vi "Obtain Request Events.vi"(8 "error in":errorcluster, 10 "Create New? (F)":bool) -> (0 "error out":errorcluster, 2 "EL72xx_DMC_ServoAxis Request Events":T1)   [LabVIEW 2023, in "EL72xx_DMC_ServoAxis.lvlib"]
doc: "This VI Obtains/Creates the Requests events that will be used for other modules to communicate with the module that owns this VI. These Requests events will be accessed only via Public API methods for this module.\n\n<b>NOTE</b>: The contents of this VI are automatically generated and modified by the <b>Tools > DQMH Consortium > DQMH</b> utilities. Consider using those utilities instead of making your own modifications to this VI.\n_____\nBased on DQMH Project Template 7.0.1.1316."
uses:
  EL72xx_DMC_ServoAxis.lvlib
  Request Events--cluster.ctl
  Stop Argument--cluster.ctl
  Show Panel Argument--cluster.ctl
  Hide Panel Argument--cluster.ctl
  Show Diagram Argument--cluster.ctl
  Get Module Execution Status Argument--cluster.ctl
  Enable_Drive Argument--cluster.ctl
  ConnectToDrive Argument--cluster.ctl
  DisconnectFromDrive Argument--cluster.ctl
  DisableDrive Argument--cluster.ctl
panel:
  # "NOTE: The contents of this VI are automatically generated and modified by the Tools > DQMH Consortium > DQMH utilities. Consider using those utilities instead of making your own modifications to this VI."
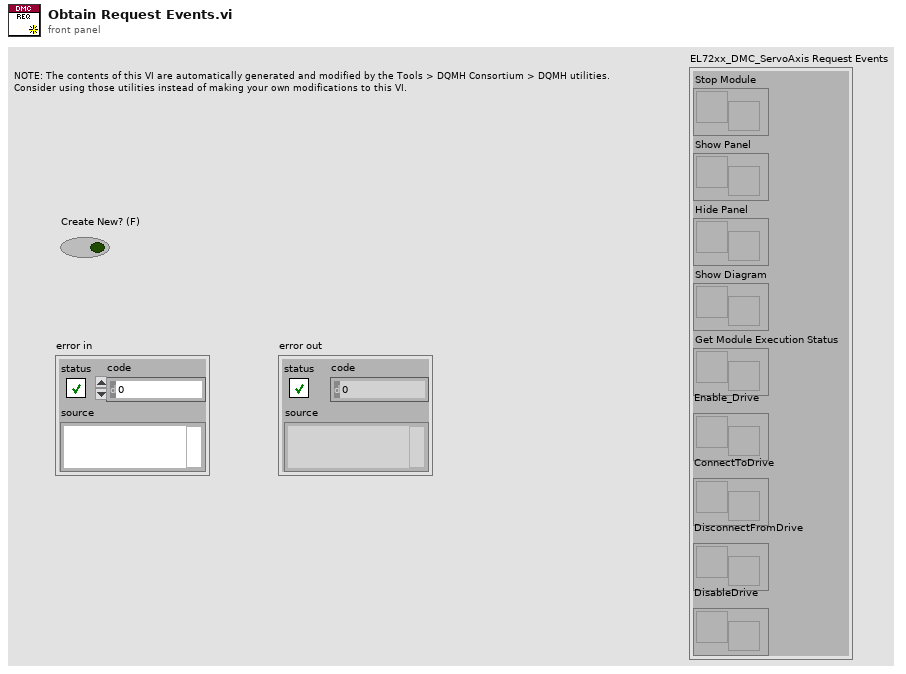
[diagram p1: front panel]
types:
  T1 = typedef "EL72xx_DMC_ServoAxis.lvlib/Request Events--cluster.ctl" = cluster{"Stop Module":refnum<user-event>, "Show Panel":refnum<user-event>, "Hide Panel":refnum<user-event>, "Show Diagram":refnum<user-event>, "Get Module Execution Status":refnum<user-event>, "Enable_Drive":refnum<user-event>, "ConnectToDrive":refnum<user-event>, "DisconnectFromDrive":refnum<user-event>, "DisableDrive":refnum<user-event>}
  T2 = typedef "EL72xx_DMC_ServoAxis.lvlib/DisableDrive Argument--cluster.ctl" = cluster{"Module ID":i32, "Disable":bool}
  T3 = typedef "EL72xx_DMC_ServoAxis.lvlib/DisconnectFromDrive Argument--cluster.ctl" = cluster{"Module ID":i32, "Boolean":bool}
  T4 = typedef "EL72xx_DMC_ServoAxis.lvlib/ConnectToDrive Argument--cluster.ctl" = cluster{"Module ID":i32, "Path":path}
  T5 = typedef "EL72xx_DMC_ServoAxis.lvlib/Enable_Drive Argument--cluster.ctl" = cluster{"Module ID":i32, "Enable":bool}
  T6 = typedef "EL72xx_DMC_ServoAxis.lvlib/Get Module Execution Status Argument--cluster.ctl" = cluster{"Module ID":i32, "Running?":bool}
  T7 = typedef "EL72xx_DMC_ServoAxis.lvlib/Show Diagram Argument--cluster.ctl" = cluster{"Module ID":i32, "Debug?":bool}
  T8 = typedef "EL72xx_DMC_ServoAxis.lvlib/Show Panel Argument--cluster.ctl" = cluster{"Module ID":i32, "Show Panel?":bool}
  T9 = typedef "EL72xx_DMC_ServoAxis.lvlib/Hide Panel Argument--cluster.ctl" = cluster{"Module ID":i32, "Hide Panel?":bool}
  T10 = typedef "EL72xx_DMC_ServoAxis.lvlib/Stop Argument--cluster.ctl" = cluster{"Module ID":i32, "Origin":string, "Exit via Stop Module Req?":bool, "Wait for Module to stop?":bool}
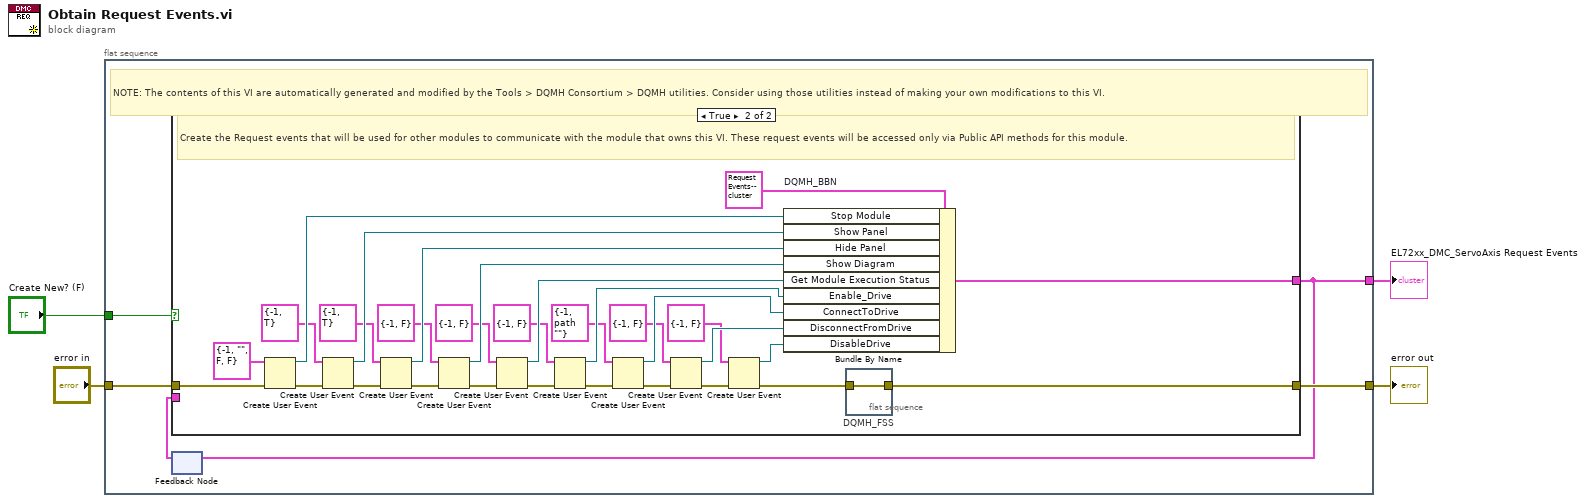
[diagram p0: block diagram]
diagram:
  n1 = flat-sequence {
    tunnel: [w9] -> w4
    tunnel: "error in" -> [w8]
    tunnel: [w6] -> w2
    tunnel: "Create New? (F)" -> [w5]
    frame #0 {
      # "NOTE: The contents of this VI are automatically generated and modified by the Tools > DQMH Consortium > DQMH utilities. Consider using those utilities instead of making your own modifications to this VI."
      n2 = feedback #1() -> (w7:T1)  [unwired: 1 in]
      n3 = case shown="True" w5 {
        tunnel: [w10 w30] -> w9
        tunnel: w8 -> [w10 w42]
        tunnel: [w11 w39] -> w6
        tunnel: w7 -> [w11 _]
        frame False {
        }
        frame True {
          # "Create the Request events that will be used for other modules to communicate with the module that owns this VI. These request events will be accessed only via Public API methods for this module."
          n4 = Create User Event(user event datatype=T10 {"Module ID"=-1, "Origin"="", "Exit via Stop Module Req?"=FALSE, "Wait for Module to stop?"=FALSE} ("Stop Argument"), error in=w42) -> (user event=w40:refnum<user-event>, error out=w37:errorcluster)
          n5 = Create User Event(user event datatype=T8 {"Module ID"=-1, "Show Panel?"=TRUE} ("Show Panel Argument"), error in=w37) -> (user event=w36:refnum<user-event>, error out=w34:errorcluster)
          n6 = Create User Event(user event datatype=T9 {"Module ID"=-1, "Hide Panel?"=TRUE} ("Hide Panel"), error in=w34) -> (user event=w33:refnum<user-event>, error out=w32:errorcluster)
          n7 = Create User Event(user event datatype=T7 {"Module ID"=-1, "Debug?"=FALSE} ("Show Diagram Argument"), error in=w32) -> (user event=w28:refnum<user-event>, error out=w29:errorcluster)
          n8 = Create User Event(user event datatype=T6 {"Module ID"=-1, "Running?"=FALSE} ("Get Module Execution Status Argument"), error in=w29) -> (user event=w25:refnum<user-event>, error out=w26:errorcluster)
          n9 = Create User Event(user event datatype=T5 {"Module ID"=-1, "Enable"=FALSE} ("Enable_Drive Argument"), error in=w26) -> (user event=w22:refnum<user-event>, error out=w23:errorcluster)
          n10 = Create User Event(user event datatype=T4 {"Module ID"=-1, "Path"=path ""} ("ConnectToDrive Argument"), error in=w23) -> (user event=w19:refnum<user-event>, error out=w20:errorcluster)
          n11 = Create User Event(user event datatype=T3 {"Module ID"=-1, "Boolean"=FALSE} ("DisconnectFromDrive Argument"), error in=w20) -> (user event=w16:refnum<user-event>, error out=w17:errorcluster)
          n12 = Create User Event(user event datatype=T2 {"Module ID"=-1, "Disable"=FALSE} ("DisableDrive Argument"), error in=w17) -> (user event=w13:refnum<user-event>, error out=w14:errorcluster)
          n13 = Bundle By Name "DQMH_BBN"(cluster=T1 {"Stop Module"=refnum, "Show Panel"=refnum, "Hide Panel"=refnum, "Show Diagram"=refnum, "Get Module Execution Status"=refnum, "Enable_Drive"=refnum, "ConnectToDrive"=refnum, "DisconnectFromDrive"=refnum, "DisableDrive"=refnum} ("output cluster"), "Stop Module"=w40, "Show Panel"=w36, "Hide Panel"=w33, "Show Diagram"=w28, "Get Module Execution Status"=w25, "Enable_Drive"=w22, "ConnectToDrive"=w19, "DisconnectFromDrive"=w16, "DisableDrive"=w13) -> (w39:T1)
          n14 = flat-sequence "DQMH_FSS" {
            tunnel: w14 -> [w43]
            tunnel: [w43] -> w30
            frame #0 {
            }
          }
        }
      }
      n15 = feedback-in #1(w6) -> ()
    }
  }
  "EL72xx_DMC_ServoAxis Request Events" <- w2
  "error out" <- w4
